vi "DCC_get_module_info.vi"(8 "Error In":errorcluster, 10 "Module No":i16 min=0 max=7 step=1, 11 "DLL Path":path) -> (0 "Error Out":errorcluster, 2 "Module No":i16, 3 "DLL Path":path, 5 "Module Info":T1)   [LabVIEW 2019]
doc: "The \"DCC_get_mode_info.vi\" gets the module serial number, card base I/O address, the slot numberr, bus number as well as the module type from the previous initialized DCC module.\nFurther, it returns whether the module specified by the module number is initialized and whether it is in use or not. \nHere the number one indicates a possible usage of the module whereas the number zero shows up if the module is already in use.\n\nAugust 2018\nFrank Quadt & Stefan Smietana\ninfo@becker-hickl.com"
uses:
  DCC_Controls/DCC_ModuleInfoCluster.ctl
panel:
  # "(c) 2018 Becker & Hickl GmbH\n     All Rights Reserved."
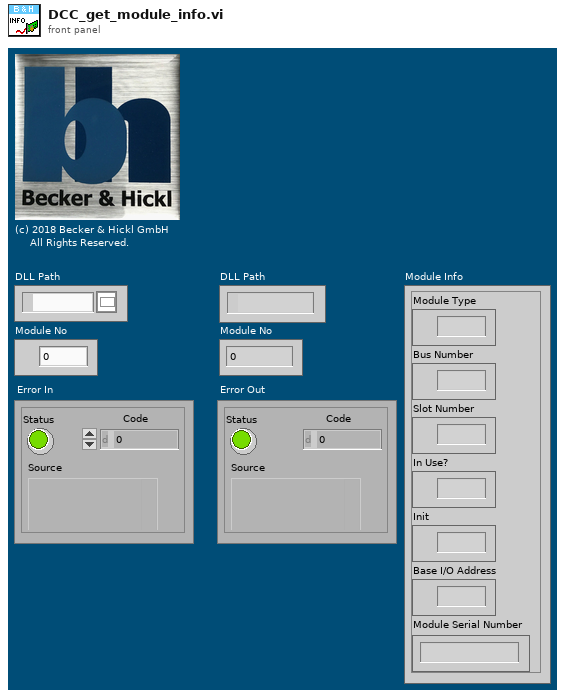
[diagram p1: front panel]
types:
  T1 = typedef "DCC_ModuleInfoCluster.ctl" = cluster{"Module Type":i16, "Bus Number":i16, "Slot Number":i16, "In Use?":i16, "Init":i16, "Base I/O Address":u16, "Module Serial Number":string}
  T2 = cluster{"[0]":u8, "[1]":u8, "[2]":u8, "[3]":u8, "[4]":u8, "[5]":u8, "[6]":u8, "[7]":u8, "[8]":u8}
  T3 = cluster{"Module Type":i16, "Bus Number":i16, "Slot Number":i16, "In Use?":i16, "Init":i16, "Base I/O Address":u16, cluster{"[0]":u8, "[1]":u8, "[2]":u8, "[3]":u8, "[4]":u8, "[5]":u8, "[6]":u8, "[7]":u8, "[8]":u8}}
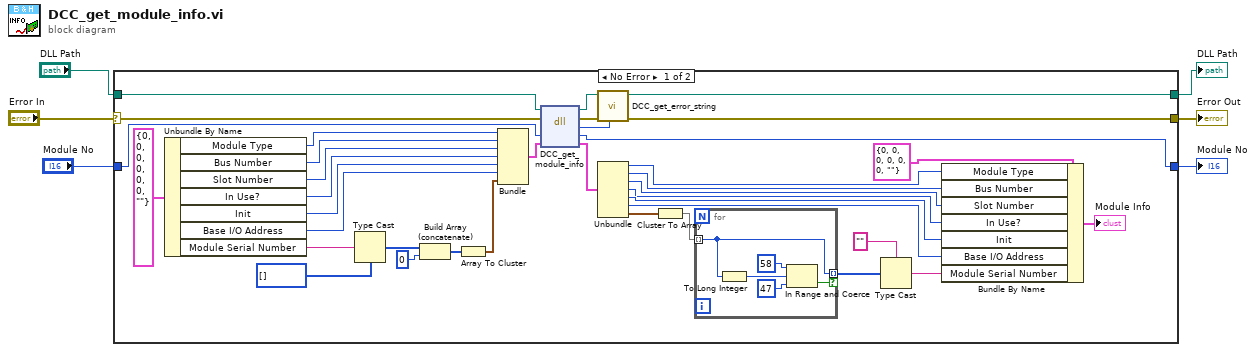
[diagram p0: block diagram]
diagram:
  n1 = case shown="No Error" "Error In" {
    selector: "Error In" -> [w43 w50]
    tunnel: [w36 w50] -> w5
    tunnel: [w37 w51] -> w4
    tunnel: "DLL Path" -> [w42 w51]
    tunnel: "Module No" -> [w41 w49]
    tunnel: [w40 w49] -> w1
    frame No Error {
      n2 = Unbundle By Name(T1 {"Module Type"=0, "Bus Number"=0, "Slot Number"=0, "In Use?"=0, "Init"=0, "Base I/O Address"=0, "Module Serial Number"=""} ("Module Info")) -> ("Module Type"=w24:i16, "Bus Number"=w23:i16, "Slot Number"=w22:i16, "In Use?"=w21:i16, "Init"=w20:i16, "Base I/O Address"=w19:u16, "Module Serial Number"=w26:string)
      n3 = Type Cast(type=u8[] [], x=w26) -> (*(type *) &x=w33:u8[])
      n4 = Build Array (concatenate)(w33, u8 0) -> (w35:u8[])
      n5 = Array To Cluster(array=w35) -> (cluster=w18:T2)
      n6 = Bundle("Module Type"=w24, "Bus Number"=w23, "Slot Number"=w22, "In Use?"=w21, "Init"=w20, "Base I/O Address"=w19, w18) -> (w25:T3)  [unwired: 1 in]
      n7 = dll-call lib="C:/Program Files/BH/DCC/DLL/dcc32.dll" fn="DCC_get_module_info"(path in=w42, error in=w43, "ModuleNo"=w41, w25) -> (path out=w38:path, error out=w39:errorcluster, "return type"=w28:i16, "ModuleNo"=w40:i16, w17:T3)  [unwired: 1 in]
      n8 = call "DCC_get_error_string.vi"("Error ID"=w28, "Error In"=w39, "DLL Path"=w38) -> ("Error Out"=w36:errorcluster, "DLL Path"=w37:path)  [unwired: 6 in, 1 out]
      n9 = Unbundle(w17) -> ("Module Type"=w11:i16, "Bus Number"=w10:i16, "Slot Number"=w9:i16, "In Use?"=w12:i16, "Init"=w13:i16, "Base I/O Address"=w14:u16, w16:T2)
      n10 = Cluster To Array(cluster=w16) -> (array=w8:u8[])
      n11 = for {
        tunnel: w8 -> [w48] mode=indexing
        tunnel: [w48] -> w7 mode=indexing if=w47
        n12 = To Long Integer(number=w48) -> (32bit integer=w46:i32)
        n13 = In Range and Coerce(upper limit=58, x=w46, lower limit=47) -> (In Range?=w47:bool)  [unwired: 1 out]
      }
      n14 = Type Cast(type="", x=w7) -> (*(type *) &x=w15:string)
      n15 = Bundle By Name(cluster=T1 {"Module Type"=0, "Bus Number"=0, "Slot Number"=0, "In Use?"=0, "Init"=0, "Base I/O Address"=0, "Module Serial Number"=""} ("Module Info"), "Module Type"=w11, "Bus Number"=w10, "Slot Number"=w9, "In Use?"=w12, "Init"=w13, "Base I/O Address"=w14, "Module Serial Number"=w15) -> (→"Module Info":T1)
    }
    frame Error {
    }
  }
  "Error Out" <- w5
  "DLL Path" <- w4
  "Module No" <- w1
